vi "Read Signal Ref.vi"(8 "error in (no error)":errorcluster, 11 "Data Saver in":refnum<class "Data Saver.lvclass">) -> (0 "error out":errorcluster, 2 "Signal Ref":refnum<vi>, 3 "Data Saver out":refnum<class "Data Saver.lvclass">)   [LabVIEW 2014, in "Data Saving.lvlib" / "Data Saver.lvclass"]
uses:
  Data Saver.lvclass
  Data Saver.lvclass/Data Saver.ctl
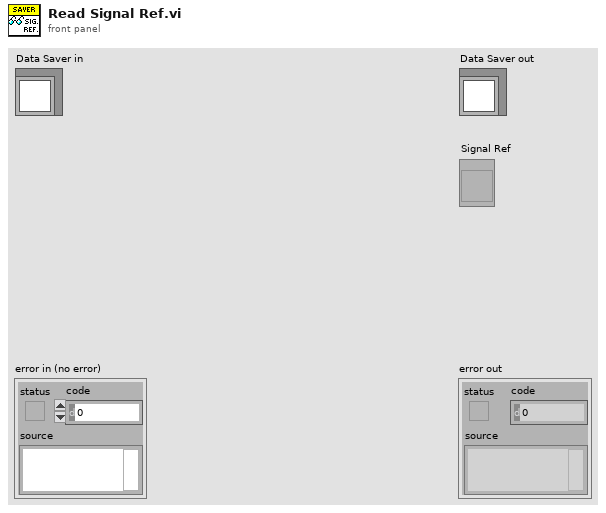
[diagram p1: front panel]
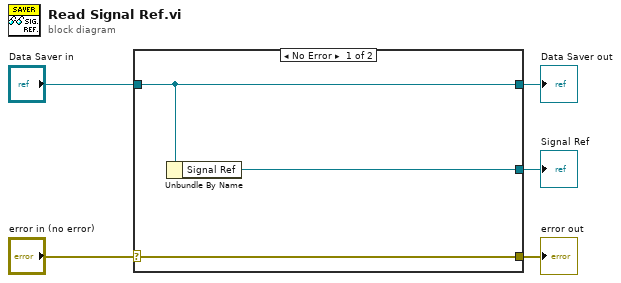
[diagram p0: block diagram]
diagram:
  n1 = case shown="No Error" "error in (no error)" {
    selector: "error in (no error)" -> [w8 w9]
    tunnel: [w8 w9] -> w4
    tunnel: [w7 w10] -> w2
    tunnel: "Data Saver in" -> [w7 w10]
    tunnel: [w6 _] -> w1
    frame No Error {
      n2 = Unbundle By Name(w7) -> ("Signal Ref"=w6:refnum<vi>)
    }
    frame Error {
    }
  }
  "error out" <- w4
  "Data Saver out" <- w2
  "Signal Ref" <- w1
